vi "File Type.vi"(8 "error in (no error)":errorcluster, 10 "File Type":u16(ring), 11 "Generador in":refnum<class "Generador.lvclass">) -> (0 "error out":errorcluster, 3 "Generador out":refnum<class "Generador.lvclass">)   [LabVIEW 2020, in "Generador señal.lvlib" / "Generador.lvclass"]
uses:
  Generador.lvclass
  C:/Program Files (x86)/National Instruments/LabVIEW 2020/vi.lib/ActorFramework/Actor/Actor.lvclass
  Generador.lvclass/Generador.ctl
  Text File/Text File/Text File.lvclass
  CSV/CSV/CSV.lvclass
  C:/Users/Asus/Dropbox/trabajos_apuntes/7 semestre/labview/Actor Framework Tarea/Text File/Text File/Text File.lvclass
  <vilib>/ActorFramework/Message Enqueuer/Message Enqueuer.lvclass/Message Enqueuer.ctl
  <vilib>/ActorFramework/Message Enqueuer/Enqueue.vi
  <vilib>/ActorFramework/Stop Msg/Stop Msg.lvclass
  C:/Program Files (x86)/National Instruments/LabVIEW 2020/vi.lib/ActorFramework/Message/Message.lvclass
  <vilib>/ActorFramework/Message Priority Queue/Priority Enqueue.vi
  <vilib>/ActorFramework/Actor/Actor.lvclass
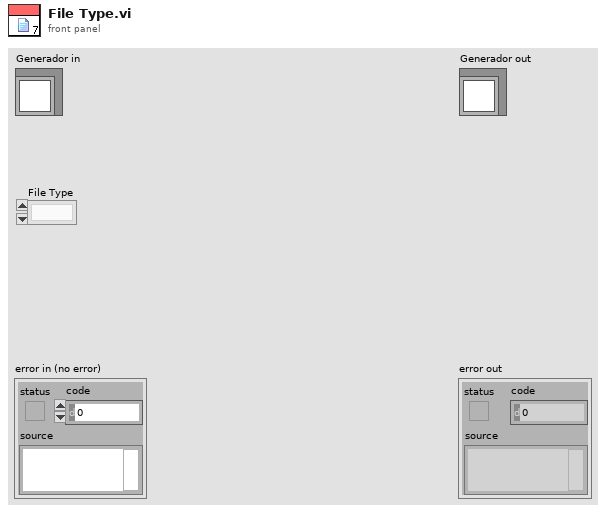
[diagram p1: front panel]
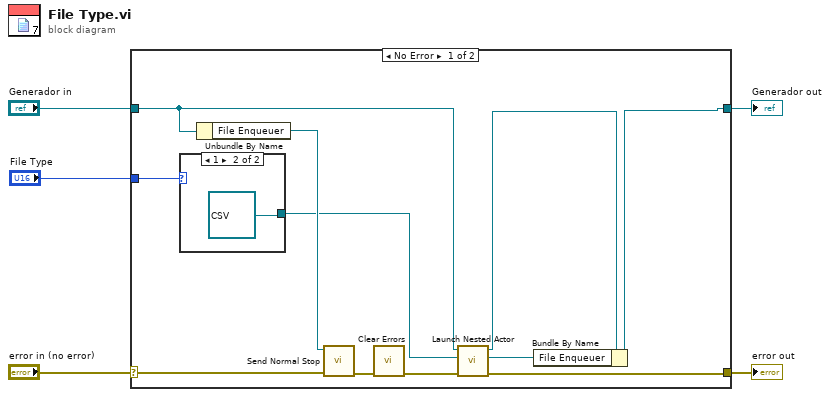
[diagram p0: block diagram]
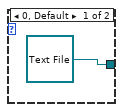
[diagram p2: hidden frame]
diagram:
  n1 = case shown="No Error" "error in (no error)" {
    selector: "error in (no error)" -> [w8 w20]
    tunnel: [w7 w20] -> w4
    tunnel: [w9 w19] -> w2
    tunnel: "Generador in" -> [w11 w19]
    tunnel: "File Type" -> [w6 _]
    frame No Error {
      n2 = case shown="1" w6 {
        tunnel: [refnum<class "Text File.lvclass"> refnum ("Text File.lvlib:Text File.lvclass") refnum<class "CSV.lvclass"> refnum ("Text File.lvlib:CSV.lvlib:CSV.lvclass")] -> w12
        frame 0, Default {
        }
        frame 1 {
        }
      }
      n3 = Unbundle By Name(w11) -> ("File Enqueuer"=w13:refnum<class "Message Enqueuer.lvclass">)
      n4 = call <vilib>:"Send Normal Stop.vi"("error in (no error)"=w8, "Message Enqueuer"=w13) -> ("error out"=w15:errorcluster)  [unwired: 9 in]
      n5 = call <vilib>:"Clear Errors.vi"("error in (no error)"=w15) -> ("error out"=w16:errorcluster)  [unwired: 5 in, 1 out]
      n6 = call <vilib>:"Launch Nested Actor.vi"("error in (no error)"=w16, "Nested Actor"=w12, "Caller Actor in"=w11) -> ("error out"=w7:errorcluster, "Nested Actor's Enqueuer"=w14:refnum<class "Message Enqueuer.lvclass">, "Caller Actor out"=w10:refnum<class "Generador.lvclass">)  [unwired: 6 in]
      n7 = Bundle By Name(cluster=w10, "File Enqueuer"=w14) -> (w9:refnum<class "Generador.lvclass">)
    }
    frame Error {
    }
  }
  "error out" <- w4
  "Generador out" <- w2
